vi "Query Temperature.vi"(8 "error in (no error)":errorcluster, 10 "Motor ID (0)":u8, 11 "Dynamixel Motor in":refnum<class "Dynamixel Motor.lvclass">) -> (0 "error out":errorcluster, 2 "Temperature (C)":u8(slide) scale=0.0..150.0, 3 "Dynamixel Motor out":refnum<class "Dynamixel Motor.lvclass">)   [LabVIEW 2016, in "Dynamixel Motor.lvclass"]
doc: "Retrieves the motor's temperature."
uses:
  <instrlib>/Dynamixel Motor/HAIOL/Dynamixel Motor.lvclass
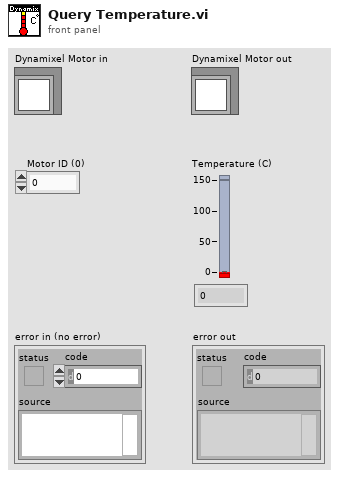
[diagram p1: front panel]
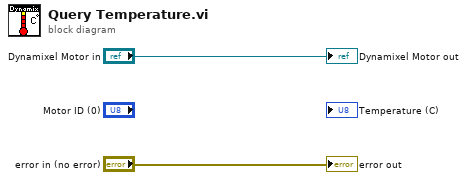
[diagram p0: block diagram]
diagram:
  "error out" <- "error in (no error)"
  "Dynamixel Motor out" <- "Dynamixel Motor in"
